vi "Instrument Manager Loop.vi"(8 "System Control":refnum<queue>, 11 "Instrument Manager":refnum<queue>) -> (0 "error out":errorcluster)   [LabVIEW 2020, in "Polar Bear Plus All-in-One Plugin.lvlib" / "Instrument Manager.lvlib"]
uses:
  Instrument Manager/Instrument Manager.lvlib
  support/Message Queue/Message Queue.lvlib
  Instrument Manager/Instrument State.ctl
  <vilib>/Utility/error.llb/Error Cluster From Error Code.vi
  <vilib>/ErrorRing/Error Ring.xnode
  Polar Bear Plus All-in-One Plugin.lvlib
  <instrlib>/RxnRover/Driver Polar Bear Plus/heater_parent/heater_parent.lvclass
  support/Message Queue/Message Cluster.ctl
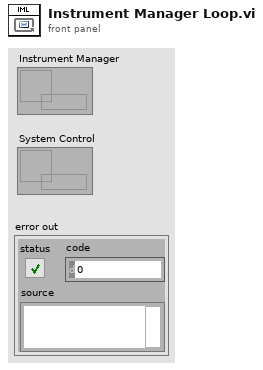
[diagram p1: front panel]
types:
  T1 = typedef "Polar Bear Plus All-in-One Plugin.lvlib/Instrument Manager.lvlib/Instrument State.ctl" = cluster{"Setpoint":dbl, "Running":bool, "Running Since":timestamp, "Data Point":cluster{"Time Stamp":timestamp, "Value":dbl}, "Sampling Rate (sec/sample)":dbl, "Ramp Rate":dbl, "Heat Switch Active?":bool, "Driver Object":refnum<class "heater_parent.lvclass">}
  T2 = cluster{"seconds since 1Jan1904":timestamp, "Current Temperature":dbl}
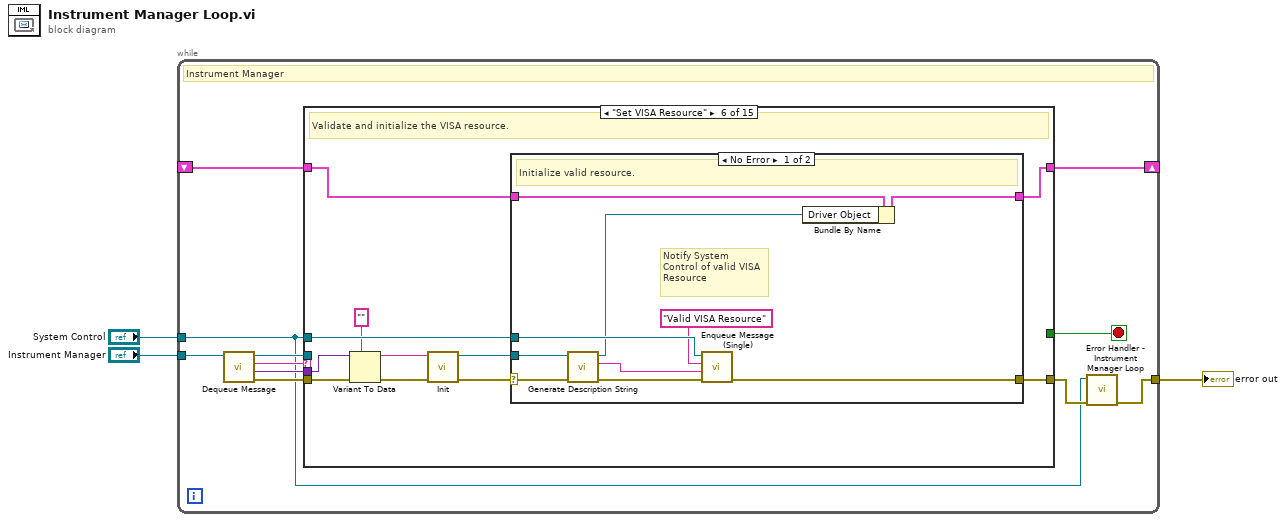
[diagram p0: block diagram]
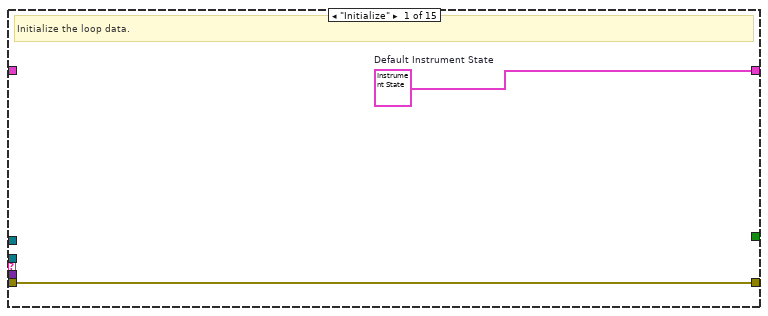
[diagram p2: hidden frame]
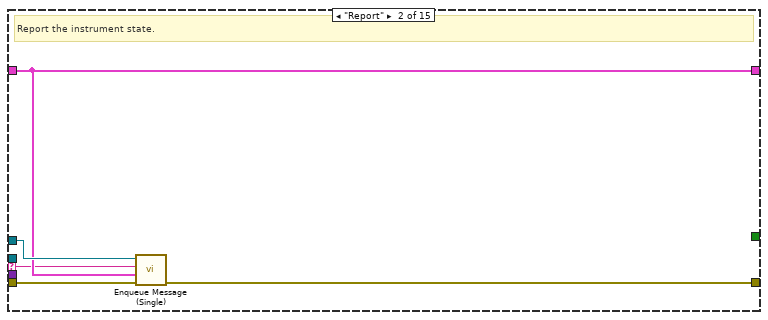
[diagram p3: hidden frame]
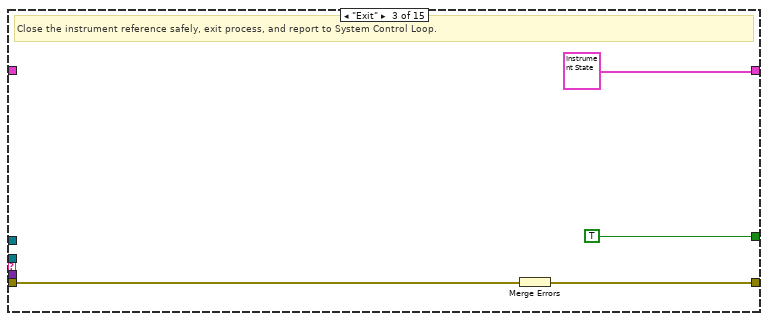
[diagram p4: hidden frame]
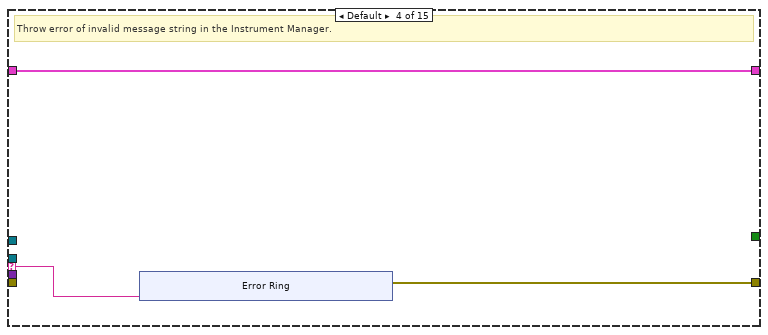
[diagram p5: hidden frame]
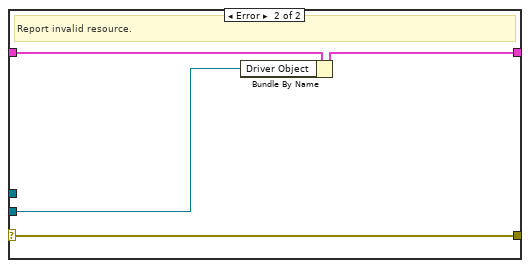
[diagram p7: hidden frame]
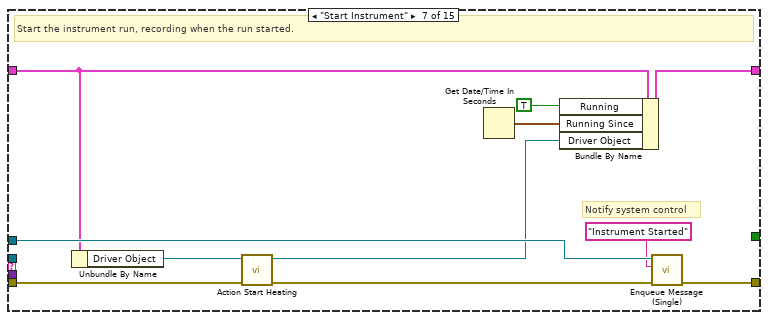
[diagram p8: hidden frame]
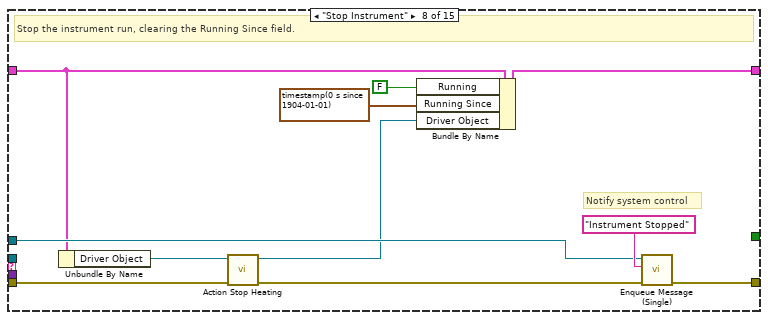
[diagram p9: hidden frame]
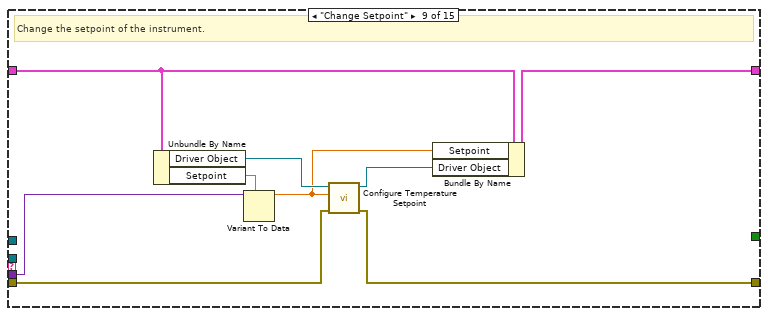
[diagram p10: hidden frame]
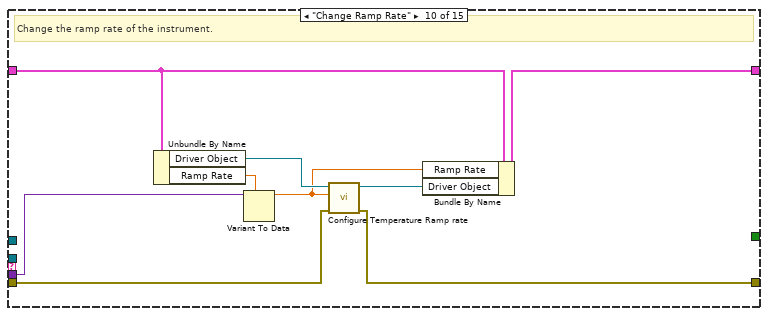
[diagram p11: hidden frame]
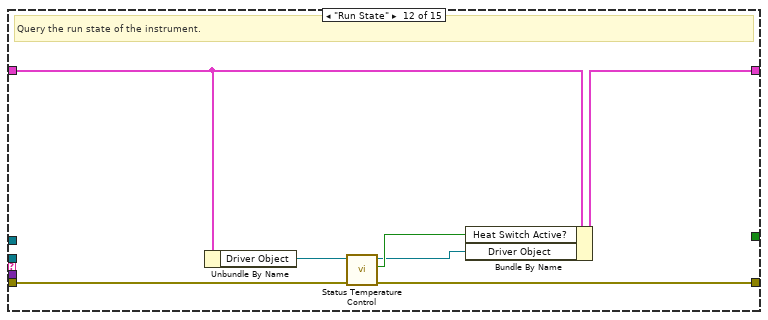
[diagram p13: hidden frame]
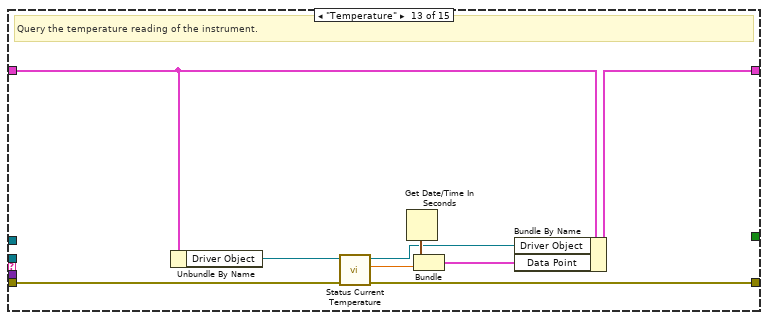
[diagram p14: hidden frame]
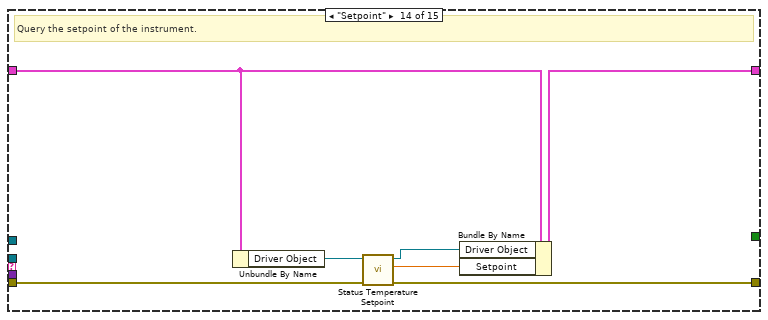
[diagram p15: hidden frame]
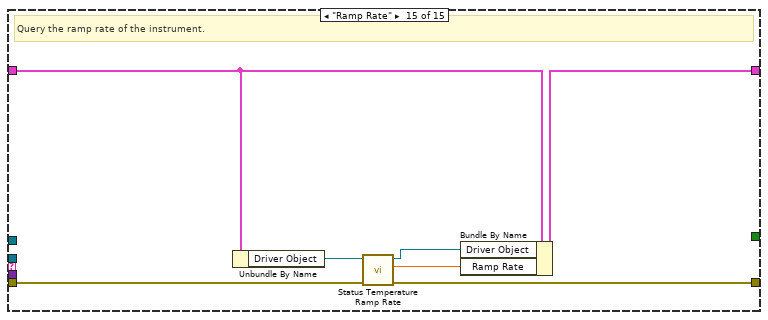
[diagram p16: hidden frame]
diagram:
  n1 = while {
    tunnel: "Instrument Manager" -> [w14]
    tunnel: "System Control" -> [w5]
    tunnel: [w8] -> w1
    shift-right: [w7] -> _
    shift-left: _ -> [w4]
    stop <- w6 stop-if-true
    # "Instrument Manager"
    n2 = call "Dequeue Message.vi"("Message Queue"=w14) -> ("error out"=w10:errorcluster, "Message Data"=w11:variant, "Message"=w13:string, "dup Message Queue"=w12:refnum<queue>)  [unwired: 7 in]
    n3 = case shown="\"Set VISA Resource\"" w13 {
      selector: w13 -> [_ w17 _ w27 _ _ _ _ _ _ _ _ _ _ _]
      tunnel: w12 -> [_ _ _ _ _ _ _ _ _ _ _ _ _ _ _]
      tunnel: w5 -> [_ w20 _ _ _ w39 w72 w82 _ _ _ _ _ _ _]
      tunnel: w11 -> [_ _ _ _ _ w45 _ _ w92 w101 _ _ _ _ _]
      tunnel: w10 -> [w16 w21 w23 _ w36 w44 w65 w77 w89 w98 w104 w111 w115 w127 w134]
      tunnel: [w16 w19 w22 w26 w36 w48 w73 w84 w88 w97 w104 w110 w114 w126 w133] -> w9
      tunnel: w4 -> [_ w18 _ w28 w37 w47 w67 w75 w91 w100 w103 w107 w117 w125 w132]
      tunnel: [w15 w18 T1 {"Setpoint"=0.0, "Running"=FALSE, "Running Since"=timestamp(0 s since 1904-01-01), "Data Point"={"Time Stamp"=timestamp(0 s since 1904-01-01), "Value"=0.0}, "Sampling Rate (sec/sample)"=0.0, "Ramp Rate"=0.0, "Heat Switch Active?"=FALSE, "Driver Object"=refnum} w28 w37 w46 w70 w81 w93 w102 w103 w108 w120 w123 w130] -> w7
      tunnel: [_ _ TRUE _ _ _ _ _ _ _ _ _ _ _ _] -> w6
      frame "Initialize" {
        w15 = T1 {"Setpoint"=0.0, "Running"=FALSE, "Running Since"=timestamp(0 s since 1904-01-01), "Data Point"={"Time Stamp"=timestamp(0 s since 1904-01-01), "Value"=0.0}, "Sampling Rate (sec/sample)"=0.0, "Ramp Rate"=0.0, "Heat Switch Active?"=FALSE, "Driver Object"=refnum}  # Default Instrument State
        # "Initialize the loop data."
      }
      frame "Report" {
        # "Report the instrument state."
        n4 = call "Enqueue Message (Single).vi"("error in (no error)"=w21, "Message Data"=w18, "Message"=w17, "Message Queue"=w20) -> ("error out"=w19:errorcluster)  [unwired: 6 in, 1 out]
      }
      frame "Exit" {
        # "Close the instrument reference safely, exit process, and report to System Control Loop."
        n5 = Merge Errors(w23) -> (w22:errorcluster)
      }
      frame Default {
        # "Throw error of invalid message string in the Instrument Manager."
        n6 = xnode "Error Ring"("parameter 0"=w27) -> ("error out"=w26:errorcluster)
      }
      frame "--- Copy This Frame ---" {
        # "Copy this frame and add responses to instrument specific messages."
      }
      frame "Set VISA Resource" {
        # "Validate and initialize the VISA resource."
        n7 = Variant To Data(error in=w44, type="", Variant=w45) -> (data=w42:string, error out=w43:errorcluster)
        n8 = call "Init.vi"("error in (no error)"=w43, "Device Descriptor in"=w42) -> ("error out"=w40:errorcluster, "PBP Driver"=w41:refnum<class "heater_parent.lvclass">)  [unwired: 8 in]
        n9 = case shown="No Error" w40 {
          selector: w40 -> [w57 w59]
          tunnel: w41 -> [w50 w60]
          tunnel: [w56 w59] -> w48
          tunnel: w47 -> [w58 w62]
          tunnel: [w53 w61] -> w46
          tunnel: w39 -> [w55 _]
          frame No Error {
            # "Notify System Control of valid VISA Resource"
            # "Initialize valid resource."
            n10 = call-dynamic "Generate Description String.vi"("error in (no error)"=w57, "heater_parent in"=w50) -> ("error out"=w52:errorcluster, "Description String"=w51:string, "heater_parent out"=w49:refnum<class "heater_parent.lvclass">)  [unwired: 7 in]
            n11 = call "Enqueue Message (Single).vi"("error in (no error)"=w52, "Message Data"=w51, "Message"="Valid VISA Resource", "Message Queue"=w55) -> ("error out"=w56:errorcluster)  [unwired: 6 in, 1 out]
            n12 = Bundle By Name(cluster=w58, "Driver Object"=w49) -> (w53:T1)
          }
          frame Error {
            # "Report invalid resource."
            n13 = Bundle By Name(cluster=w62, "Driver Object"=w60) -> (w61:T1)
          }
        }
      }
      frame "Start Instrument" {
        # "Notify system control"
        # "Start the instrument run, recording when the run started."
        n14 = Unbundle By Name(w67) -> ("Driver Object"=w66:refnum<class "heater_parent.lvclass">)
        n15 = call-dynamic "Action Start Heating.vi"("error in (no error)"=w65, "heater_parent in"=w66) -> ("error out"=w64:errorcluster, "heater_parent out"=w63:refnum<class "heater_parent.lvclass">)  [unwired: 8 in]
        n16 = Get Date/Time In Seconds() -> (seconds since 1Jan1904=w68:timestamp)
        n17 = Bundle By Name(cluster=w67, "Running"=TRUE, "Running Since"=w68, "Driver Object"=w63) -> (w70:T1)
        n18 = call "Enqueue Message (Single).vi"("error in (no error)"=w64, "Message"="Instrument Started", "Message Queue"=w72) -> ("error out"=w73:errorcluster)  [unwired: 7 in, 1 out]
      }
      frame "Stop Instrument" {
        # "Notify system control"
        # "Stop the instrument run, clearing the Running Since field."
        n19 = Unbundle By Name(w75) -> ("Driver Object"=w78:refnum<class "heater_parent.lvclass">)
        n20 = call-dynamic "Action Stop Heating.vi"("error in (no error)"=w77, "heater_parent in"=w78) -> ("error out"=w76:errorcluster, "heater_parent out"=w74:refnum<class "heater_parent.lvclass">)  [unwired: 8 in]
        n21 = Bundle By Name(cluster=w75, "Running"=FALSE, "Running Since"=timestamp(0 s since 1904-01-01), "Driver Object"=w74) -> (w81:T1)
        n22 = call "Enqueue Message (Single).vi"("error in (no error)"=w76, "Message"="Instrument Stopped", "Message Queue"=w82) -> ("error out"=w84:errorcluster)  [unwired: 7 in, 1 out]
      }
      frame "Change Setpoint" {
        # "Change the setpoint of the instrument."
        n23 = Unbundle By Name(w91) -> ("Driver Object"=w87:refnum<class "heater_parent.lvclass">, "Setpoint"=w90:dbl)
        n24 = Variant To Data(type=w90, Variant=w92) -> (data=w86:dbl)  [unwired: 1 in, 1 out]
        n25 = call-dynamic "Configure Temperature Setpoint.vi"("error in (no error)"=w89, "New Setpoint"=w86, "heater_parent in"=w87) -> ("error out"=w88:errorcluster, "heater_parent out"=w85:refnum<class "heater_parent.lvclass">)  [unwired: 7 in]
        n26 = Bundle By Name(cluster=w91, "Setpoint"=w86, "Driver Object"=w85) -> (w93:T1)
      }
      frame "Change Ramp Rate" {
        # "Change the ramp rate of the instrument."
        n27 = Unbundle By Name(w100) -> ("Driver Object"=w96:refnum<class "heater_parent.lvclass">, "Ramp Rate"=w99:dbl)
        n28 = Variant To Data(type=w99, Variant=w101) -> (data=w95:dbl)  [unwired: 1 in, 1 out]
        n29 = call-dynamic "Configure Temperature Ramp rate.vi"("error in (no error)"=w98, "New Ramp Rate"=w95, "heater_parent in"=w96) -> ("error out"=w97:errorcluster, "heater_parent out"=w94:refnum<class "heater_parent.lvclass">)  [unwired: 7 in]
        n30 = Bundle By Name(cluster=w100, "Ramp Rate"=w95, "Driver Object"=w94) -> (w102:T1)
      }
      frame "--- Copy for Get State Messages ---" {
        # "#CodeNeeded - Use the Bundle by Name function to bundle the new state value into the Instrument State cluster."
        # "#CodeNeeded - Add instrument driver call to query the instrument state requested"
        # "Duplicate this case for messages cases that will query the instrument state."
      }
      frame "Run State" {
        # "Query the run state of the instrument."
        n31 = Unbundle By Name(w107) -> ("Driver Object"=w109:refnum<class "heater_parent.lvclass">)
        n32 = call-dynamic "Status Temperature Control.vi"("error in (no error)"=w111, "heater_parent in"=w109) -> ("error out"=w110:errorcluster, "Heating or cooling on?"=w106:bool, "heater_parent out"=w105:refnum<class "heater_parent.lvclass">)  [unwired: 7 in]
        n33 = Bundle By Name(cluster=w107, "Heat Switch Active?"=w106, "Driver Object"=w105) -> (w108:T1)
      }
      frame "Temperature" {
        # "Query the temperature reading of the instrument."
        n34 = Unbundle By Name(w117) -> ("Driver Object"=w116:refnum<class "heater_parent.lvclass">)
        n35 = call-dynamic "Status Current Temperature.vi"("error in (no error)"=w115, "heater_parent in"=w116) -> ("error out"=w114:errorcluster, "Current Temperature"=w113:dbl, "heater_parent out"=w112:refnum<class "heater_parent.lvclass">)  [unwired: 7 in]
        n36 = Get Date/Time In Seconds() -> (seconds since 1Jan1904=w119:timestamp)
        n37 = Bundle("seconds since 1Jan1904"=w119, "Current Temperature"=w113) -> (w118:T2)  [unwired: 1 in]
        n38 = Bundle By Name(cluster=w117, "Driver Object"=w112, "Data Point"=w118) -> (w120:T1)
      }
      frame "Setpoint" {
        # "Query the setpoint of the instrument."
        n39 = Unbundle By Name(w125) -> ("Driver Object"=w124:refnum<class "heater_parent.lvclass">)
        n40 = call-dynamic "Status Temperature Setpoint.vi"("error in (no error)"=w127, "heater_parent in"=w124) -> ("error out"=w126:errorcluster, "Setpoint"=w122:dbl, "heater_parent out"=w121:refnum<class "heater_parent.lvclass">)  [unwired: 7 in]
        n41 = Bundle By Name(cluster=w125, "Driver Object"=w121, "Setpoint"=w122) -> (w123:T1)
      }
      frame "Ramp Rate" {
        # "Query the ramp rate of the instrument."
        n42 = Unbundle By Name(w132) -> ("Driver Object"=w131:refnum<class "heater_parent.lvclass">)
        n43 = call-dynamic "Status Temperature Ramp Rate.vi"("error in (no error)"=w134, "heater_parent in"=w131) -> ("error out"=w133:errorcluster, "Ramp Rate"=w129:dbl, "heater_parent out"=w128:refnum<class "heater_parent.lvclass">)  [unwired: 7 in]
        n44 = Bundle By Name(cluster=w132, "Driver Object"=w128, "Ramp Rate"=w129) -> (w130:T1)
      }
    }
    n45 = call "Error Handler - Instrument Manager Loop.vi"("error in (no error)"=w9, "Message Queue"=w5) -> ("dup error in"=w8:errorcluster)  [unwired: 8 in, 1 out]
  }
  "error out" <- w1
